vi "Open Hardware.vi"(8 "error in (no error)":errorcluster, 11 "Inst.Attocube-3DR in":refnum<class "Inst.Attocube-3DR.lvclass">) -> (0 "error out":errorcluster, 3 "Inst.Attocube-3DR out":refnum<class "Inst.Attocube-3DR.lvclass">)   [LabVIEW 2019, in "Inst.Attocube-3DR.lvclass"]
uses:
  Inst.Attocube-3DR.lvclass
  Inst.Attocube-3DR.lvclass/Inst.Attocube-3DR.ctl
  <userlib>/LevyLab/Instrument Framework/Instrument/Instrument.lvclass
  drivers/ANC350.lvlib
  C:/Program Files (x86)/National Instruments/LabVIEW 2019/user.lib/LevyLab/Instrument Framework/Instrument/Instrument.lvclass
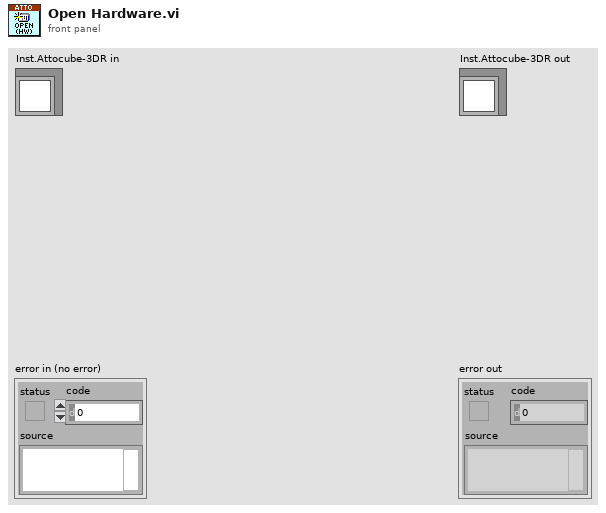
[diagram p1: front panel]
types:
  T1 = cluster{"error ":bool, "error number":i32, "error code":string}
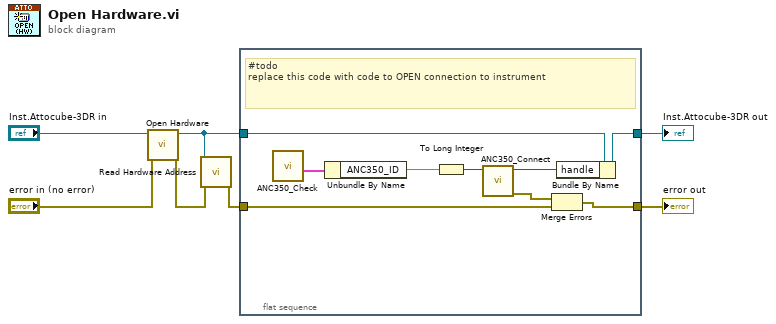
[diagram p0: block diagram]
diagram:
  n1 = call-parent "Open Hardware.vi"("error in (no error)"="error in (no error)", "Instrument in"="Inst.Attocube-3DR in") -> ("error out"=w5:errorcluster, "Instrument out"=w4:refnum<class "Inst.Attocube-3DR.lvclass">)  [unwired: 8 in]
  n2 = call <userlib>:"Read Hardware Address.vi"("error in (no error)"=w5, "Instrument in"=w4) -> ("error out"=w2:errorcluster)  [unwired: 7 in, 2 out]
  n3 = flat-sequence {
    tunnel: w4 -> [w16]
    tunnel: [w15] -> w3
    tunnel: w2 -> [w11]
    tunnel: [w9] -> w1
    frame #0 {
      # "#todo\nreplace this code with code to OPEN connection to instrument"
      n4 = call "ANC350_Check.vi"() -> ("ANC350_Status"=w13:cluster{"ANC350_ID":dbl, "locked":bool})  [unwired: 6 in, 1 out]
      n5 = Unbundle By Name(w13) -> ("ANC350_ID"=w8:dbl)
      n6 = To Long Integer(number=w8) -> (32bit integer=w12:i32)
      n7 = call "ANC350_Connect.vi"("device no"=w12) -> ("error out"=w10:T1, "handle"=w14:i32)  [unwired: 5 in]
      n8 = Merge Errors(w10, w11) -> (w9:errorcluster)
      n9 = Bundle By Name(cluster=w16, "handle"=w14) -> (w15:refnum<class "Inst.Attocube-3DR.lvclass">)
    }
  }
  "error out" <- w1
  "Inst.Attocube-3DR out" <- w3
